vi "BRig_Host__Loop_Consumer_dataRTwrite__getType.vi"(11 "input_data_RTwrite":string) -> (2 "output_type":u8, 3 "output_data_RT_write":string)   [LabVIEW 2014]
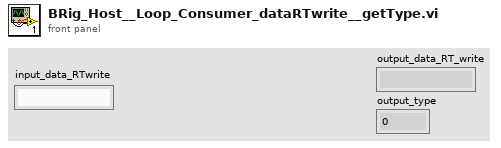
[diagram p1: front panel]
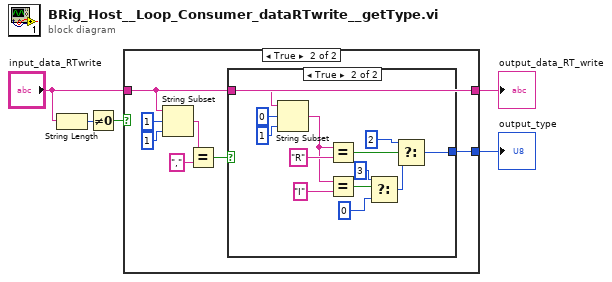
[diagram p0: block diagram]
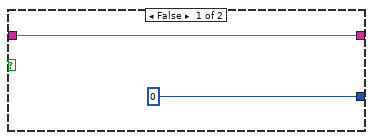
[diagram p2: hidden frame]
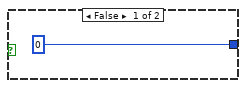
[diagram p3: hidden frame]
diagram:
  n1 = String Length(string="input_data_RTwrite") -> (length=w5:i32)
  n2 = Not Equal To 0?(x=w5) -> (x != 0?=w4:bool)
  n3 = case shown="True" w4 {
    tunnel: "input_data_RTwrite" -> [w7 w11]
    tunnel: [w7 w11] -> w2
    tunnel: [u8 0 w14] -> w1
    frame False {
    }
    frame True {
      n4 = String Subset(string=w11, offset (0)=1, length (rest)=1 ("length (rest)")) -> (substring=w10:string)
      n5 = Equal?(x=w10, y=",") -> (x = y?=w9:bool)
      n6 = case shown="True" w9 {
        tunnel: w11 -> [_ w17]
        tunnel: [u8 0 w16] -> w14
        frame False {
        }
        frame True {
          n7 = String Subset(string=w17, offset (0)=0, length (rest)=1 ("length (rest)")) -> (substring=w18:string)
          n8 = Equal?(x=w18, y="R") -> (x = y?=w19:bool)
          n9 = Equal?(x=w18, y="I") -> (x = y?=w24:bool)
          n10 = Select(t=u8 3, s=w24, f=u8 0) -> (s? t:f=w21:u8)
          n11 = Select(t=u8 2, s=w19, f=w21) -> (s? t:f=w16:u8)
        }
      }
    }
  }
  "output_data_RT_write" <- w2
  "output_type" <- w1
